vi "HFG_Core.vi"(7 "HFG Commands":T3=enum."Initialize", 8 "Error In":errorcluster, 9 "Heartbeat state IN":T1=enum."Completed", 10 "VI Name (Calling VIs name by default)":string) -> (0 "Error Out":errorcluster, 1 "All States":cluster{string[], T1[]}, 2 "Heartbeat Event":refnum<user-event>, 3 "Heartbeat Data OUT":T2={"Heartbeat state"=enum."Completed", "VI Name"=""})   [LabVIEW 2012]
doc: "SciScan 1.2 160622\nThis FGV is used to generate heartbeat events used for inter process communication within the project.\n\nA heartbeat event is created when the module writes its 'Run State' to the FGV. The event can be listened by other sections of the program for a status update\n\nNote that automatic error handling has been disabled in this VI (due to undesirable application shutdown behaviour) - Error handling to be implemented by the user\nTips:\n-----\n1. To set the status of a VI, run a 'Set' case with either the VI name or VI reference"
uses:
  Custom Controls and Typedefs/HFG Commands.ctl
  Custom Controls/Heartbeat_States.ctl
  Custom Controls/Heartbeat Event Structure.ctl
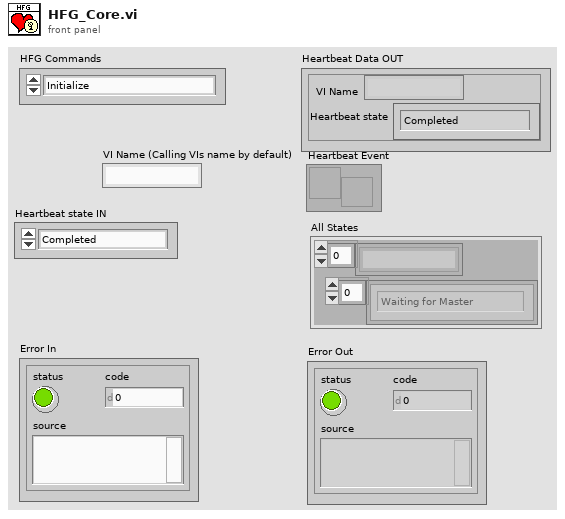
[diagram p1: front panel]
types:
  T1 = typedef "Heartbeat_States.ctl" = enum16{"Waiting for Master", "Instruction Issued", "Waiting for Slave Completion", "Completed", "Cancelled", "Failed", "Broken Link"}
  T2 = typedef "Heartbeat Event Structure.ctl" = cluster{"Heartbeat state":T1, "VI Name":string}
  T3 = typedef "HFG Commands.ctl" = enum16{"Set", "Get", "Initialize"}
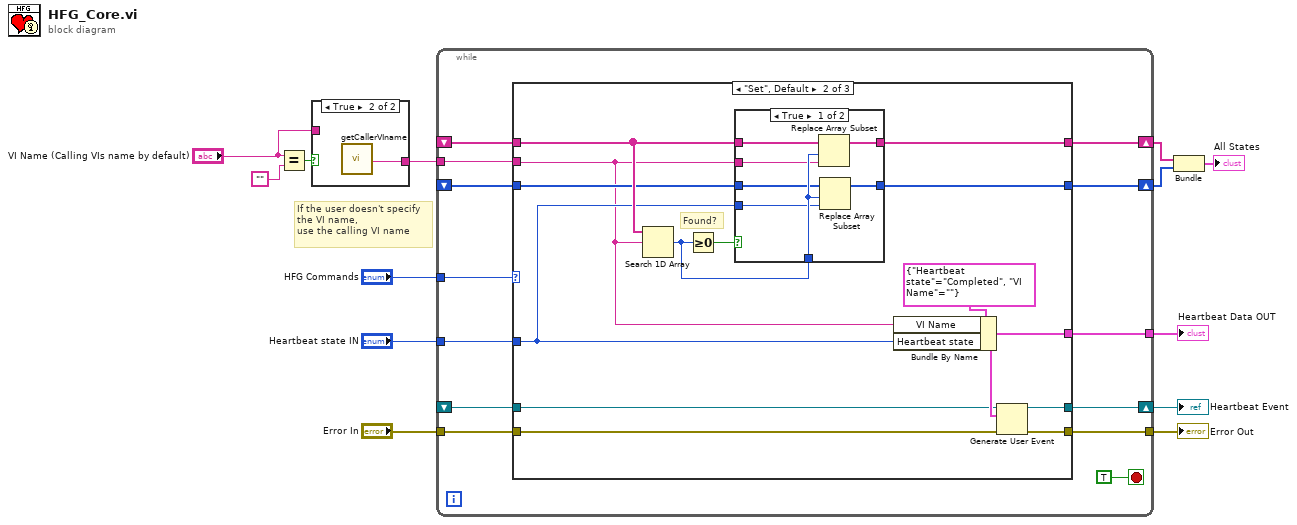
[diagram p0: block diagram]
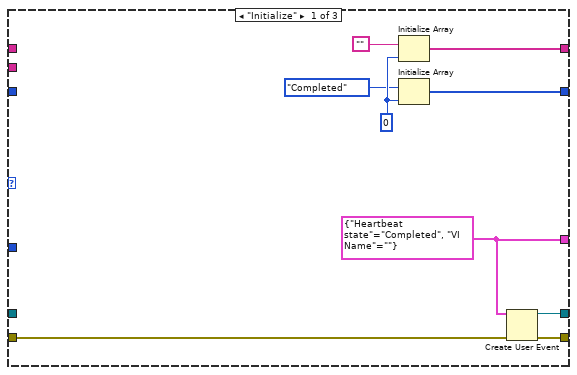
[diagram p3: hidden frame]
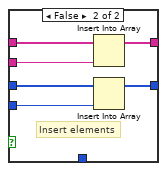
[diagram p4: hidden frame]
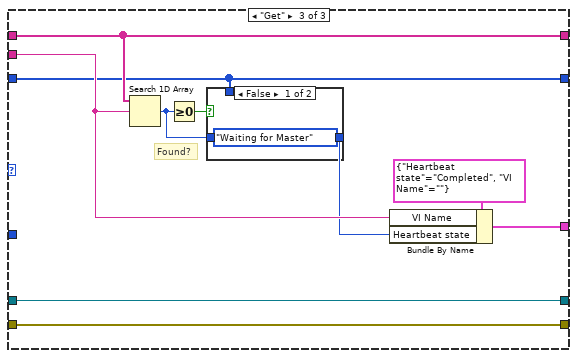
[diagram p5: hidden frame]
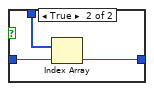
[diagram p6: hidden frame]
diagram:
  # "If the user doesn't specify\nthe VI name,\nuse the calling VI name"
  n1 = Equal?(x="VI Name (Calling VIs name by default)", y="") -> (x = y?=w3:bool)
  n2 = case shown="True" w3 {
    tunnel: [w14 w15] -> w2
    tunnel: "VI Name (Calling VIs name by default)" -> [w14 _]
    frame False {
    }
    frame True {
      n3 = call "getCallerVIname.vi"() -> ("VI name"=w15:string)  [unwired: 19 in]
    }
  }
  n4 = while {
    tunnel: "HFG Commands" -> [w28]
    shift-right: [w26] -> w8
    shift-left: _ -> [w25]
    tunnel: w2 -> [w24]
    shift-right: [w22] -> w9
    shift-left: _ -> [w21]
    shift-right: [w19] -> w7
    shift-left: _ -> [w18]
    tunnel: "Heartbeat state IN" -> [w17]
    tunnel: [w16] -> w10
    tunnel: "Error In" -> [w23]
    tunnel: [w20] -> w12
    stop <- TRUE stop-if-true
    n5 = case shown="\"Set\", Default" w28 {
      tunnel: [w36 w45 w70] -> w26
      tunnel: w25 -> [_ w50 w70]
      tunnel: w24 -> [_ w38 w69]
      tunnel: w23 -> [w32 w49 w72]
      tunnel: [w30 w48 w71] -> w22
      tunnel: w21 -> [_ w39 w71]
      tunnel: [w31 w47 w72] -> w20
      tunnel: [w33 w42 w66] -> w19
      tunnel: w18 -> [_ w43 w66]
      tunnel: w17 -> [_ w41 _]
      tunnel: [w29 w40 w73] -> w16
      frame "Initialize" {
        w29 = T2 {"Heartbeat state"=enum."Completed", "VI Name"=""} ("Heartbeat Event")
        w35 = 0 ("dimension size")
        n6 = Initialize Array("", w35) -> (w36:string[])
        n7 = Initialize Array(Heartbeat_States."Completed" ("Run state Input"), w35) -> (w33:T1[])
        n8 = Create User Event(user event datatype=w29, error in=w32) -> (user event=w30:refnum<user-event>, error out=w31:errorcluster)
      }
      frame "Set", Default {
        # "Found?"
        n9 = Search 1D Array(1D array=w50, element=w38) -> (index of element=w46:i32)  [unwired: 1 in]
        n10 = Greater Or Equal To 0?(x=w46) -> (x >= 0?=w51:bool)
        n11 = case shown="True" w51 {
          tunnel: w50 -> [w58 w64]
          tunnel: w38 -> [w55 w62]
          tunnel: w46 -> [w56 _]
          tunnel: [w57 w63] -> w45
          tunnel: w43 -> [w54 w61]
          tunnel: w41 -> [w53 w60]
          tunnel: [w52 w59] -> w42
          frame True {
            n12 = Replace Array Subset(array=w58, new element=w55, index=w56) -> (w57:string[])
            n13 = Replace Array Subset(array=w54, new element=w53, index=w56) -> (w52:T1[])
          }
          frame False {
            # "Insert elements"
            n14 = Insert Into Array(array=w64, new element=w62) -> (w63:string[])  [unwired: 1 in]
            n15 = Insert Into Array(array=w61, new element=w60) -> (w59:T1[])  [unwired: 1 in]
          }
        }
        n16 = Bundle By Name(cluster=T2 {"Heartbeat state"=enum."Completed", "VI Name"=""} ("Heartbeat Event"), "VI Name"=w38, "Heartbeat state"=w41) -> (w40:T2)
        n17 = Generate User Event(user event=w39, event data cluster=w40, error in=w49) -> (user event out=w48:refnum<user-event>, error out=w47:errorcluster)
      }
      frame "Get" {
        # "Found?"
        n18 = Search 1D Array(1D array=w70, element=w69) -> (index of element=w67:i32)  [unwired: 1 in]
        n19 = Greater Or Equal To 0?(x=w67) -> (x >= 0?=w68:bool)
        n20 = case shown="False" w68 {
          tunnel: w67 -> [_ w77]
          tunnel: w66 -> [_ w78]
          tunnel: [Heartbeat_States."Waiting for Master" ("Run state Input") w76] -> w65
          frame False {
          }
          frame True {
            n21 = Index Array(array=w78, index=w77) -> (element=w76:T1)
          }
        }
        n22 = Bundle By Name(cluster=T2 {"Heartbeat state"=enum."Completed", "VI Name"=""} ("Heartbeat Event"), "VI Name"=w69, "Heartbeat state"=w65) -> (w73:T2)
      }
    }
  }
  "Error Out" <- w12
  "Heartbeat Data OUT" <- w10
  "Heartbeat Event" <- w9
  n23 = Bundle(w8, w7) -> (→"All States":cluster{string[], T1[]})  [unwired: 1 in]
